vi "TCPGetVariableSets.vi"(1 "error in (no error)":errorcluster, 4 "connection ID":refnum<k5>) -> ()   [LabVIEW 2013]
uses:
  FBVarSet.ctl
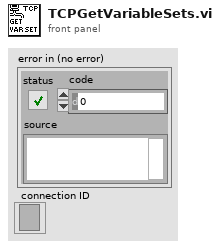
[diagram p1: front panel]
types:
  T1 = typedef "FBVarSet.ctl" = cluster{"DoubleVars":cluster{"Name":string, "Value":dbl}[], "StrVars":cluster{"Name":string, "Value":string}[]}
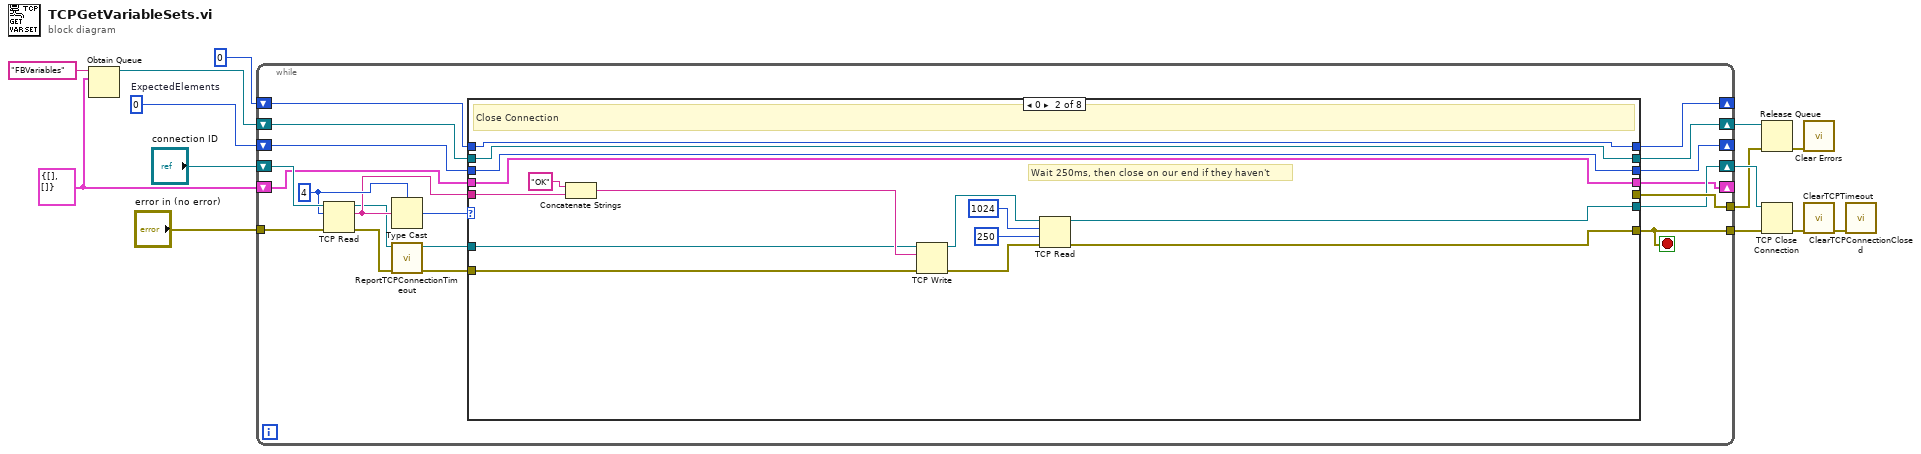
[diagram p0: block diagram]
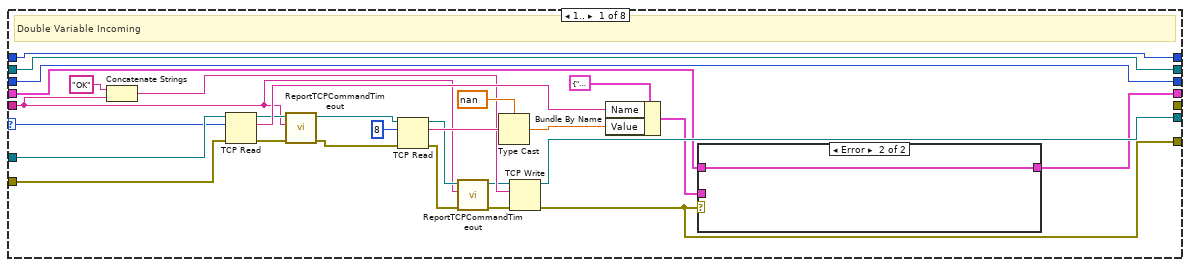
[diagram p2: hidden frame]
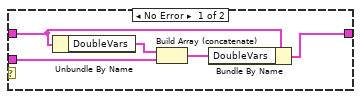
[diagram p3: hidden frame]
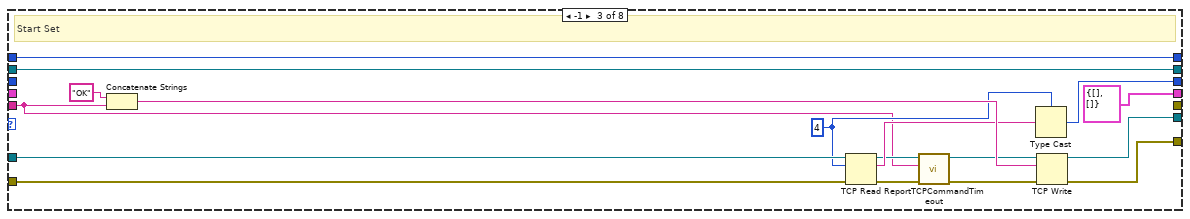
[diagram p4: hidden frame]
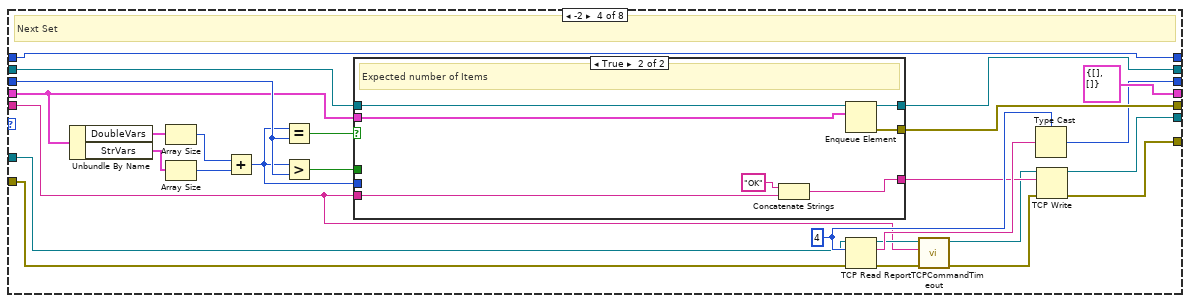
[diagram p5: hidden frame]
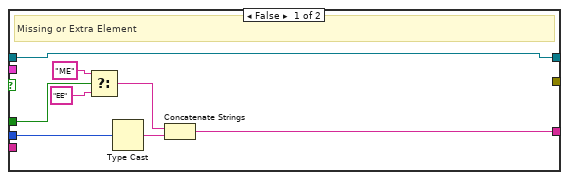
[diagram p6: hidden frame]
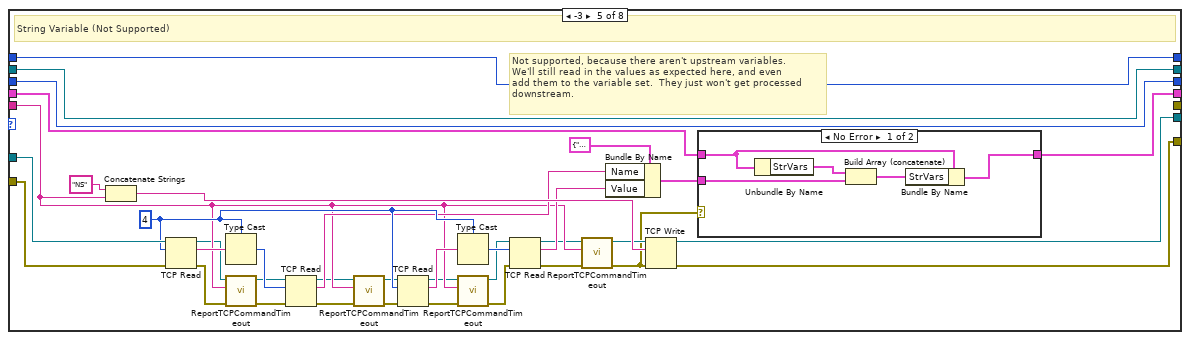
[diagram p7: hidden frame]
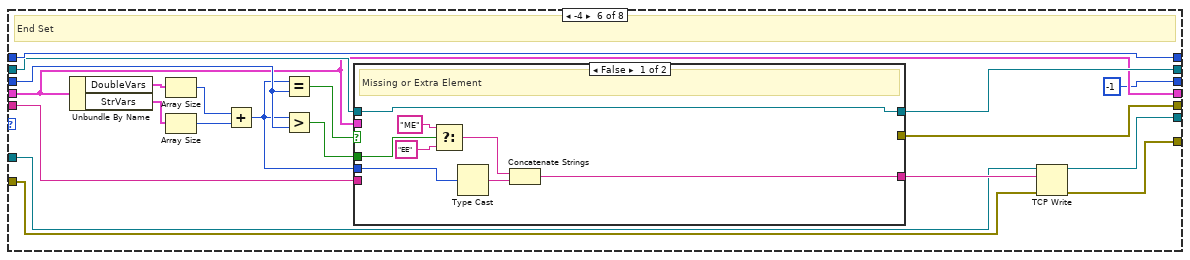
[diagram p9: hidden frame]
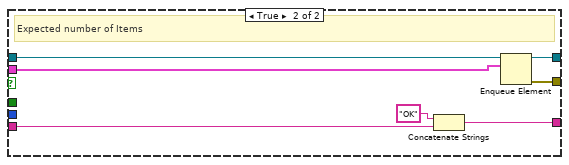
[diagram p10: hidden frame]
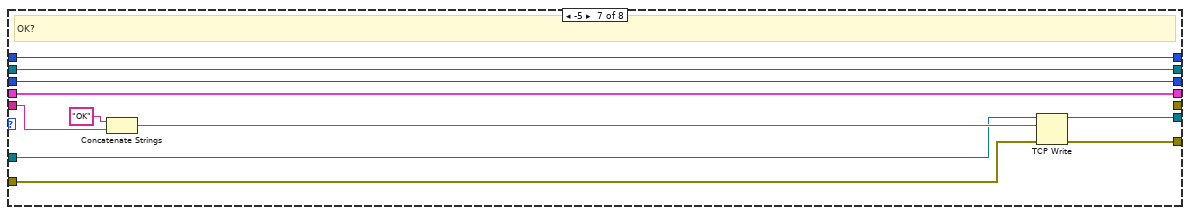
[diagram p11: hidden frame]
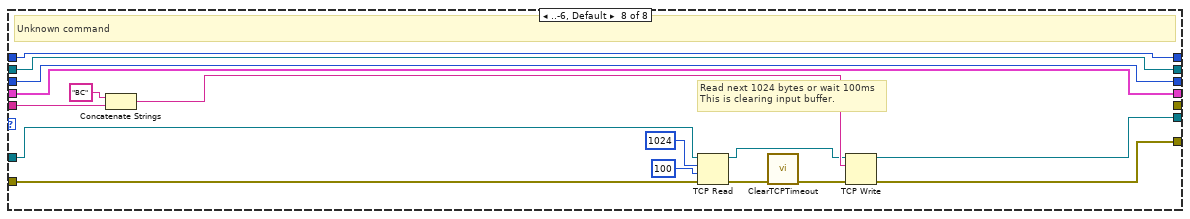
[diagram p12: hidden frame]
diagram:
  w4 = 0  # ExpectedElements
  w3 = T1 {"DoubleVars"=[], "StrVars"=[]} ("VarSet")
  n1 = Obtain Queue(name (unnamed)="FBVariables", element data type=w3) -> (queue out=w9:refnum<queue>)  [unwired: 3 in, 2 out]
  n2 = while {
    tunnel: [w24] -> w14
    shift-right: [w23] -> w13
    shift-left: "connection ID" -> [w34]
    tunnel: "error in (no error)" -> [w32]
    shift-right: [w26] -> w8
    shift-left: w9 -> [w27]
    tunnel: [w25] -> w7
    shift-right: [w29] -> _
    shift-left: 0 -> [w30]
    shift-right: [w21] -> _
    shift-left: w3 -> [w22]
    shift-right: [w19] -> _
    shift-left: w4 -> [w20]
    stop <- w24 stop-if-true
    w33 = 4
    n3 = TCP Read(connection ID=w34, bytes to read=w33, error in (no error)=w32) -> (connection ID out=w16:refnum<k5>, data out=w28:string, error out=w18:errorcluster)  [unwired: 2 in]
    n4 = Type Cast(type=w33, x=w28) -> (*(type *) &x=w31:i32)
    n5 = call "ReportTCPConnectionTimeout.vi"("error in (no error)"=w18, "connection ID"=w16) -> ("error out"=w17:errorcluster, "connection ID out"=w15:refnum<k5>)  [unwired: 8 in]
    n6 = case shown="0" w31 {
      selector: w31 -> [w58 _ _ _ _ _ _ _]
      tunnel: w30 -> [w62 w70 w100 w127 w171 w205 w223 w234]
      tunnel: [w62 w70 w100 w127 w171 w205 w223 w234] -> w29
      tunnel: w28 -> [w36 w83 w84 w101 w159 w196 w231 w247]
      tunnel: w15 -> [w59 w76 w92 w109 w173 w186 w221 w240]
      tunnel: w17 -> [w60 w77 w93 w113 w174 w187 w222 w241]
      tunnel: w27 -> [w61 w81 w99 w117 w178 w195 w229 w245]
      tunnel: [w61 w81 w99 w116 w178 w194 w229 w245] -> w26
      tunnel: [_ _ _ w114 _ w193 _ _] -> w25
      tunnel: [w35 w69 w95 w106 w177 w190 w228 w244] -> w24
      tunnel: [w54 w74 w94 w107 w175 w191 w226 w242] -> w23
      tunnel: w22 -> [w52 w71 _ w115 w165 w189 w225 w236]
      tunnel: [w53 w71 T1 {"DoubleVars"=[], "StrVars"=[]} ("VarSet") T1 {"DoubleVars"=[], "StrVars"=[]} ("VarSet") w164 w189 w225 w236] -> w21
      tunnel: w20 -> [w47 w72 _ w121 w172 w199 w224 w235]
      tunnel: [w47 w72 w89 w110 w172 -1 ("ExpectedElements") w224 w235] -> w19
      frame 1.. {
        # "Double Variable Incoming"
        n7 = Concatenate Strings("OK" ("string"), w36) -> (w46:string)
        n8 = TCP Read(connection ID=w59, bytes to read=w58, error in (no error)=w60) -> (connection ID out=w41:refnum<k5>, data out=w50:string, error out=w44:errorcluster)  [unwired: 2 in]
        n9 = call "ReportTCPCommandTimeout.vi"("error in (no error)"=w44, "command"=w36, "connection ID"=w41) -> ("error out"=w43:errorcluster, "connection ID out"=w42:refnum<k5>)  [unwired: 7 in]
        n10 = TCP Read(connection ID=w42, bytes to read=8, error in (no error)=w43) -> (connection ID out=w37:refnum<k5>, data out=w56:string, error out=w40:errorcluster)  [unwired: 2 in]
        n11 = call "ReportTCPCommandTimeout.vi"("error in (no error)"=w40, "command"=w36, "connection ID"=w37) -> ("error out"=w39:errorcluster, "connection ID out"=w38:refnum<k5>)  [unwired: 7 in]
        n12 = Type Cast(type=nan, x=w56) -> (*(type *) &x=w49:dbl)
        n13 = TCP Write(connection ID=w38, data in=w46, error in (no error)=w39) -> (connection ID out=w54:refnum<k5>, error out=w35:errorcluster)  [unwired: 1 in, 1 out]
        n14 = Bundle By Name(cluster=cluster{"Name":string, "Value":dbl} {"Name"="", "Value"=0.0} ("element"), "Name"=w50, "Value"=w49) -> (w48:cluster{"Name":string, "Value":dbl})
        n15 = case shown="Error" w35 {
          tunnel: [w67 w68] -> w53
          tunnel: w52 -> [w66 w68]
          tunnel: w48 -> [w63 _]
          frame No Error {
            n16 = Unbundle By Name(w66) -> ("DoubleVars"=w64:cluster{"Name":string, "Value":dbl}[])
            n17 = Build Array (concatenate)(w64, w63) -> (w65:cluster{"Name":string, "Value":dbl}[])
            n18 = Bundle By Name(cluster=w66, "DoubleVars"=w65) -> (w67:T1)
          }
          frame Error {
          }
        }
      }
      frame 0 {
        # "Wait 250ms, then close on our end if they haven't"
        # "Close Connection"
        n19 = Concatenate Strings("OK" ("string"), w83) -> (w80:string)
        n20 = TCP Write(connection ID=w76, data in=w80, error in (no error)=w77) -> (connection ID out=w75:refnum<k5>, error out=w73:errorcluster)  [unwired: 1 in, 1 out]
        n21 = TCP Read(connection ID=w75, bytes to read=1024, error in (no error)=w73, 9:250 ("timeout ms (25000)")) -> (connection ID out=w74:refnum<k5>, error out=w69:errorcluster)  [unwired: 1 in, 1 out]
      }
      frame -1 {
        w90 = 4 ("bytes to read")
        # "Start Set"
        n22 = Concatenate Strings("OK" ("string"), w84) -> (w96:string)
        n23 = TCP Read(connection ID=w92, bytes to read=w90, error in (no error)=w93) -> (connection ID out=w85:refnum<k5>, data out=w91:string, error out=w88:errorcluster)  [unwired: 2 in]
        n24 = call "ReportTCPCommandTimeout.vi"("error in (no error)"=w88, "command"=w84, "connection ID"=w85) -> ("error out"=w87:errorcluster, "connection ID out"=w86:refnum<k5>)  [unwired: 7 in]
        n25 = Type Cast(type=w90, x=w91) -> (*(type *) &x=w89:i32)
        n26 = TCP Write(connection ID=w86, data in=w96, error in (no error)=w87) -> (connection ID out=w94:refnum<k5>, error out=w95:errorcluster)  [unwired: 1 in, 1 out]
      }
      frame -2 {
        w111 = 4
        # "Next Set"
        n27 = Unbundle By Name(w115) -> ("DoubleVars"=w126:cluster{"Name":string, "Value":dbl}[], "StrVars"=w125:cluster{"Name":string, "Value":string}[])
        n28 = Array Size(array=w126) -> (size(s)=w124:i32)
        n29 = Array Size(array=w125) -> (size(s)=w123:i32)
        n30 = Add(x=w124, y=w123) -> (x+y=w118:i32)
        n31 = Equal?(x=w118, y=w121) -> (x = y?=w122:bool)
        n32 = Greater?(x=w118, y=w121) -> (0:w120:bool)
        n33 = case shown="True" w122 {
          tunnel: w120 -> [w130 _]
          tunnel: w118 -> [w135 _]
          tunnel: w101 -> [_ w138]
          tunnel: w117 -> [w128 w142]
          tunnel: [w128 w141] -> w116
          tunnel: w115 -> [_ w140]
          tunnel: [_ w139] -> w114
          tunnel: [w129 w136] -> w108
          frame False {
            # "Missing or Extra Element"
            n34 = Select(t="ME" ("name (unnamed)"), s=w130, f="EE" ("name (unnamed)")) -> (s? t:f=w133:string)
            n35 = Type Cast(x=w135) -> (*(type *) &x=w134:string)  [unwired: 1 in]
            n36 = Concatenate Strings(w133, w134) -> (w129:string)
          }
          frame True {
            # "Expected number of Items"
            n37 = Concatenate Strings("OK" ("string"), w138) -> (w136:string)
            n38 = Enqueue Element(queue=w142, element=w140) -> (queue out=w141:refnum<queue>, error out=w139:errorcluster)  [unwired: 2 in, 1 out]
          }
        }
        n39 = TCP Read(connection ID=w109, bytes to read=w111, error in (no error)=w113) -> (connection ID out=w102:refnum<k5>, data out=w112:string, error out=w105:errorcluster)  [unwired: 2 in]
        n40 = call "ReportTCPCommandTimeout.vi"("error in (no error)"=w105, "command"=w101, "connection ID"=w102) -> ("error out"=w104:errorcluster, "connection ID out"=w103:refnum<k5>)  [unwired: 7 in]
        n41 = Type Cast(type=w111, x=w112) -> (*(type *) &x=w110:i32)
        n42 = TCP Write(connection ID=w103, data in=w108, error in (no error)=w104) -> (connection ID out=w107:refnum<k5>, error out=w106:errorcluster)  [unwired: 1 in, 1 out]
      }
      frame -3 {
        w166 = 4 ("bytes to read")
        # "Not supported, because there aren't upstream variables.\nWe'll still read in the values as expected here, and even\nadd them to the variable set.  They just won't get processed\ndownstream."
        # "String Variable (Not Supported)"
        n43 = Concatenate Strings("NS" ("string"), w159) -> (w176:string)
        n44 = TCP Read(connection ID=w173, bytes to read=w166, error in (no error)=w174) -> (connection ID out=w151:refnum<k5>, data out=w170:string, error out=w153:errorcluster)  [unwired: 2 in]
        n45 = Type Cast(type=w166, x=w170) -> (*(type *) &x=w169:i32)
        n46 = call "ReportTCPCommandTimeout.vi"("error in (no error)"=w153, "command"=w159, "connection ID"=w151) -> ("error out"=w152:errorcluster, "connection ID out"=w150:refnum<k5>)  [unwired: 7 in]
        n47 = TCP Read(connection ID=w150, bytes to read=w169, error in (no error)=w152) -> (connection ID out=w149:refnum<k5>, data out=w162:string, error out=w155:errorcluster)  [unwired: 2 in]
        n48 = call "ReportTCPCommandTimeout.vi"("error in (no error)"=w155, "command"=w159, "connection ID"=w149) -> ("error out"=w154:errorcluster, "connection ID out"=w148:refnum<k5>)  [unwired: 7 in]
        n49 = TCP Read(connection ID=w148, bytes to read=w166, error in (no error)=w154) -> (connection ID out=w147:refnum<k5>, data out=w167:string, error out=w157:errorcluster)  [unwired: 2 in]
        n50 = Type Cast(type=w166, x=w167) -> (*(type *) &x=w168:i32)
        n51 = call "ReportTCPCommandTimeout.vi"("error in (no error)"=w157, "command"=w159, "connection ID"=w147) -> ("error out"=w156:errorcluster, "connection ID out"=w146:refnum<k5>)  [unwired: 7 in]
        n52 = TCP Read(connection ID=w146, bytes to read=w168, error in (no error)=w156) -> (connection ID out=w145:refnum<k5>, data out=w161:string, error out=w158:errorcluster)  [unwired: 2 in]
        n53 = call "ReportTCPCommandTimeout.vi"("error in (no error)"=w158, "command"=w159, "connection ID"=w145) -> ("error out"=w143:errorcluster, "connection ID out"=w144:refnum<k5>)  [unwired: 7 in]
        n54 = Bundle By Name(cluster=cluster{"Name":string, "Value":string} {"Name"="", "Value"=""} ("StrVar"), "Name"=w162, "Value"=w161) -> (w160:cluster{"Name":string, "Value":string})
        n55 = TCP Write(connection ID=w144, data in=w176, error in (no error)=w143) -> (connection ID out=w175:refnum<k5>, error out=w177:errorcluster)  [unwired: 1 in, 1 out]
        n56 = case shown="No Error" w143 {
          tunnel: w165 -> [w184 w185]
          tunnel: [w183 w185] -> w164
          tunnel: w160 -> [w180 _]
          frame No Error {
            n57 = Unbundle By Name(w184) -> ("StrVars"=w182:cluster{"Name":string, "Value":string}[])
            n58 = Build Array (concatenate)(w182, w180) -> (w181:cluster{"Name":string, "Value":string}[])
            n59 = Bundle By Name(cluster=w184, "StrVars"=w181) -> (w183:T1)
          }
          frame Error {
          }
        }
      }
      frame -4 {
        # "End Set"
        n60 = Unbundle By Name(w189) -> ("DoubleVars"=w204:cluster{"Name":string, "Value":dbl}[], "StrVars"=w203:cluster{"Name":string, "Value":string}[])
        n61 = Array Size(array=w204) -> (size(s)=w202:i32)
        n62 = Array Size(array=w203) -> (size(s)=w201:i32)
        n63 = Add(x=w202, y=w201) -> (x+y=w197:i32)
        n64 = Equal?(x=w197, y=w199) -> (x = y?=w200:bool)
        n65 = Greater?(x=w197, y=w199) -> (0:w198:bool)
        n66 = case shown="False" w200 {
          tunnel: w198 -> [w208 _]
          tunnel: w197 -> [w213 _]
          tunnel: w196 -> [_ w216]
          tunnel: w195 -> [w206 w220]
          tunnel: [w206 w219] -> w194
          tunnel: w189 -> [_ w218]
          tunnel: [_ w217] -> w193
          tunnel: [w207 w214] -> w192
          frame False {
            # "Missing or Extra Element"
            n67 = Select(t="ME" ("name (unnamed)"), s=w208, f="EE" ("name (unnamed)")) -> (s? t:f=w211:string)
            n68 = Type Cast(x=w213) -> (*(type *) &x=w212:string)  [unwired: 1 in]
            n69 = Concatenate Strings(w211, w212) -> (w207:string)
          }
          frame True {
            # "Expected number of Items"
            n70 = Concatenate Strings("OK" ("string"), w216) -> (w214:string)
            n71 = Enqueue Element(queue=w220, element=w218) -> (queue out=w219:refnum<queue>, error out=w217:errorcluster)  [unwired: 2 in, 1 out]
          }
        }
        n72 = TCP Write(connection ID=w186, data in=w192, error in (no error)=w187) -> (connection ID out=w191:refnum<k5>, error out=w190:errorcluster)  [unwired: 1 in, 1 out]
      }
      frame -5 {
        # "OK?"
        n73 = Concatenate Strings("OK" ("string"), w231) -> (w227:string)
        n74 = TCP Write(connection ID=w221, data in=w227, error in (no error)=w222) -> (connection ID out=w226:refnum<k5>, error out=w228:errorcluster)  [unwired: 1 in, 1 out]
      }
      frame ..-6, Default {
        # "Read next 1024 bytes or wait 100ms\nThis is clearing input buffer."
        # "Unknown command"
        n75 = Concatenate Strings("BC" ("string"), w247) -> (w243:string)
        n76 = TCP Read(connection ID=w240, bytes to read=1024, error in (no error)=w241, 9:100 ("timeout ms (25000)")) -> (connection ID out=w239:refnum<k5>, error out=w233:errorcluster)  [unwired: 1 in, 1 out]
        n77 = call "ClearTCPTimeout.vi"("error in (no error)"=w233) -> ("error out"=w232:errorcluster)  [unwired: 9 in, 1 out]
        n78 = TCP Write(connection ID=w239, data in=w243, error in (no error)=w232) -> (connection ID out=w242:refnum<k5>, error out=w244:errorcluster)  [unwired: 1 in, 1 out]
      }
    }
  }
  n79 = Release Queue(queue=w8, error in (no error)=w7) -> (error out=w6:errorcluster)  [unwired: 1 in, 2 out]
  n80 = TCP Close Connection(connection ID=w13, error in (no error)=w14) -> (error out=w2:errorcluster)  [unwired: 1 in, 1 out]
  n81 = call <vilib>:"Clear Errors.vi"("error in (no error)"=w6) -> ()  [unwired: 6 in, 1 out]
  n82 = call "ClearTCPTimeout.vi"("error in (no error)"=w2) -> ("error out"=w1:errorcluster)  [unwired: 9 in, 1 out]
  n83 = call "ClearTCPConnectionClosed.vi"("error in (no error)"=w1) -> ()  [unwired: 9 in, 2 out]
